vi "Connect.vi"(8 "error in":errorcluster, 11 "IMG_SRC in":refnum<class "IMG_SRC.lvclass">) -> (0 "error out":errorcluster, 3 "IMG_SRC out":refnum<class "IMG_SRC.lvclass">)   [LabVIEW 2018, in "IMG_SRC.lvlib" / "IMG_SRC.lvclass"]
uses:
  IMG_SRC.lvclass
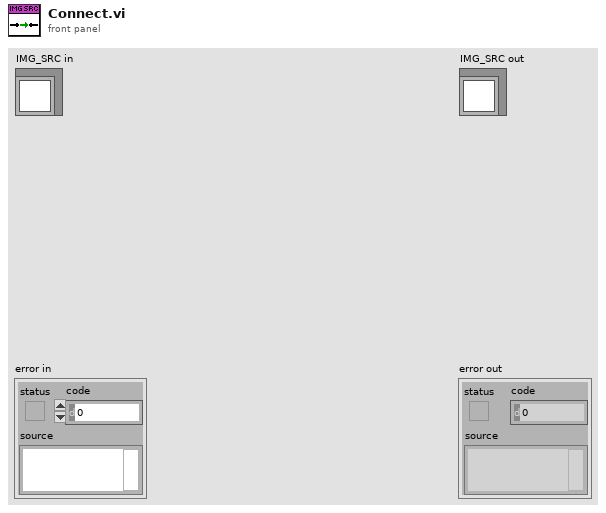
[diagram p1: front panel]
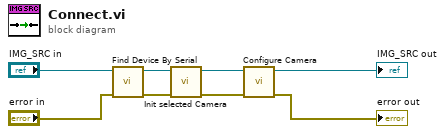
[diagram p0: block diagram]
diagram:
  n1 = call "Find Device By Serial.vi"("error in"="error in", "IMG_SRC in"="IMG_SRC in") -> ("error out"=w7:errorcluster, "IMG_SRC out"=w8:refnum<class "IMG_SRC.lvclass">)  [unwired: 8 in]
  n2 = call "Init selected Camera.vi"("error in"=w7, "IMG_SRC in"=w8) -> ("error out"=w4:errorcluster, "IMG_SRC out"=w3:refnum<class "IMG_SRC.lvclass">)  [unwired: 8 in]
  n3 = call "Configure Camera.vi"("error in"=w4, "IMG_SRC in"=w3) -> ("error out"=→"error out":errorcluster, "IMG_SRC out"=→"IMG_SRC out":refnum<class "IMG_SRC.lvclass">)  [unwired: 8 in]
